vi "FreerunMultiple.vi"(7 "speeds":dbl[](array[numeric]), 8 "error in (no error)":errorcluster, 9 "taskId":i32(ring) items=["TLibrary", "T01", "T02", "T03", "T04", "T05", "T06", "T07", "T08", "T09", "T10", "T11", "T12", "T13", "T14", "T15", "T16", "T17", "T18", "T19", "T20", "T21", "T22", "T23", "T24", "T25", "T26", "T27", "T28", "T29", "T30", "T31"], 10 "axis names":string[](array[string]), 11 "controller in":refnum<k24>) -> (0 "error out":errorcluster, 3 "controller out":refnum<k24>)   [LabVIEW 2018, in "Aerotech.lvlib"]
uses:
  Aerotech.lvlib
  C:/Program Files (x86)/Aerotech/A3200/LabVIEW/2010/Bin/Aerotech.A3200.dll
  Program Files (x86)/Aerotech/A3200/LabVIEW/2010/Bin/Aerotech.A3200.dll
  C:/Users/HEP/Documents/GitHub/UCSB-Gantry-HEP-2018/Drivers/Aerotech A3200/Bin/Aerotech.A3200.LabVIEW.dll
  UCSB-Gantry-HEP-2018/Drivers/Aerotech A3200/Bin/Aerotech.A3200.LabVIEW.dll
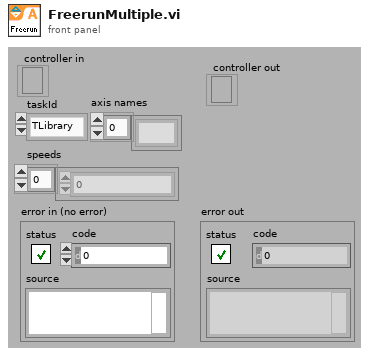
[diagram p1: front panel]
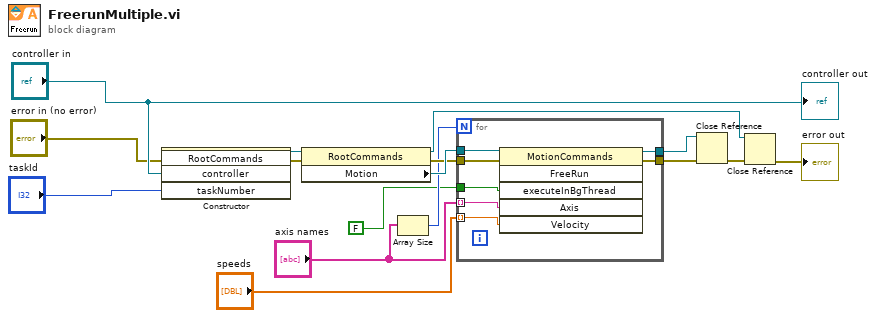
[diagram p0: block diagram]
diagram:
  n1 = constructor class="RootCommands"(error in="error in (no error)", "controller"="controller in", "taskNumber"="taskId") -> (reference out=w11:refnum<k24>, error out=w10:errorcluster)  [unwired: 2 in, 3 out]
  n2 = property class="RootCommands"(reference=w11, error in=w10) -> (reference out=w6:refnum<k24>, error out=w12:errorcluster, "Motion"=w13:refnum<k24>)
  n3 = Array Size(array="axis names") -> (size(s)=w3:i32)
  n4 = for {
    N: w3 -> [_]
    tunnel: FALSE ("return immediately") -> [w23]
    tunnel: w13 -> [w22]
    tunnel: w12 -> [w21]
    tunnel: [w20] -> w9
    tunnel: [w19] -> w8
    tunnel: "axis names" -> [w18] mode=indexing
    tunnel: "speeds" -> [w17] mode=indexing
    n5 = invoke class="MotionCommands" method="FreeRun"(reference=w22, error in=w21, "executeInBgThread"=w23, "Axis"=w18, "Velocity"=w17) -> (reference out=w19:refnum<k24>, error out=w20:errorcluster)  [unwired: 1 in, 4 out]
  }
  n6 = Close Reference(reference=w8, error in (no error)=w9) -> (error out=w7:errorcluster)
  n7 = Close Reference(reference=w6, error in (no error)=w7) -> (error out=→"error out":errorcluster)
  "controller out" <- "controller in"
